vi "Analyze_Data.vi"(8 "error in (no error)":errorcluster, 9 "Number of Samples":dbl, 11 "Data In":dbl[](array[numeric])) -> (0 "error out":errorcluster)   [LabVIEW 2024]
uses:
  <vilib>/Analysis/2dsp.llb/Real FFT.vi
  <vilib>/Analysis/NI_AALPro.lvlib
  <vilib>/Analysis/NI_AALBase.lvlib
panel:
  in  "Copy Graph Data (Mag)":bool
  in  "Copy Graph Data (Phase)":bool
  out "Phase Spectrum":dbl[](graph) caption="Magnitude Spectrum"
  in  "Copy Graph Phase":bool
  in  "Copy Graph (Mag)":bool
  out "Amplitude":string
  out "Frequency (Hz)":string
  in  "Annotate List Cluster":T1
  in  "Show Labels":bool
  in  "Voltage Analysis":bool
  out "Output 2":string
  out "Output":string
  in  "FFT Analysis":bool
  in  "Statistic Analysis":bool
  out "Magnitude Spectrum":dbl[](graph)
  # "Frequency Peaks:"
  # "Frequency (Hz)"
  # "Amplitude"
  # "F0\nF1\nF2"
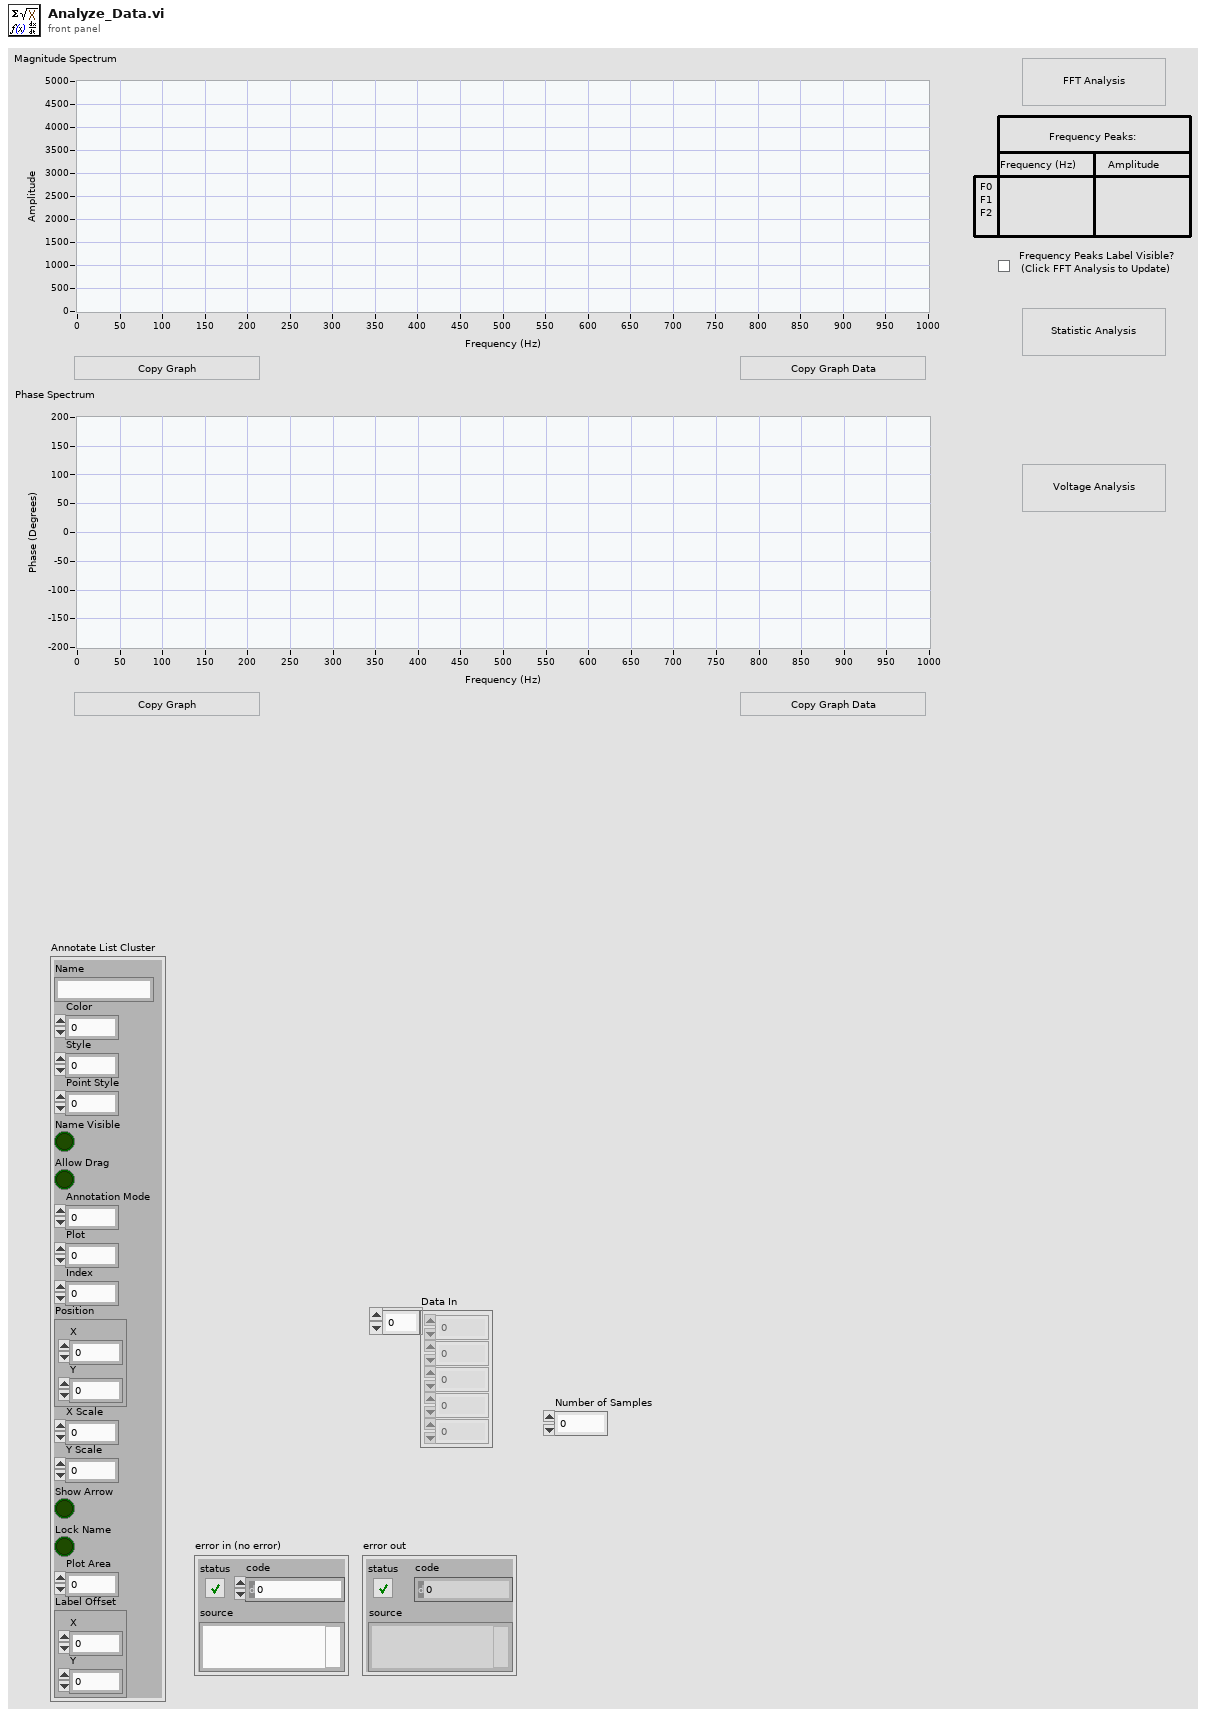
[diagram p1: front panel]
types:
  T1 = cluster{"Name":string, "Color":u32, "Style":u8, "Point Style":u8, "Name Visible":bool, "Allow Drag":bool, "Annotation Mode":u32, "Plot":i32, "Index":i32, "Position":cluster{"X":dbl, "Y":dbl}, "X Scale":u32, "Y Scale":u32, "Show Arrow":bool, "Lock Name":bool, "Plot Area":i32, "Label Offset":cluster{"X":dbl, "Y":dbl}}
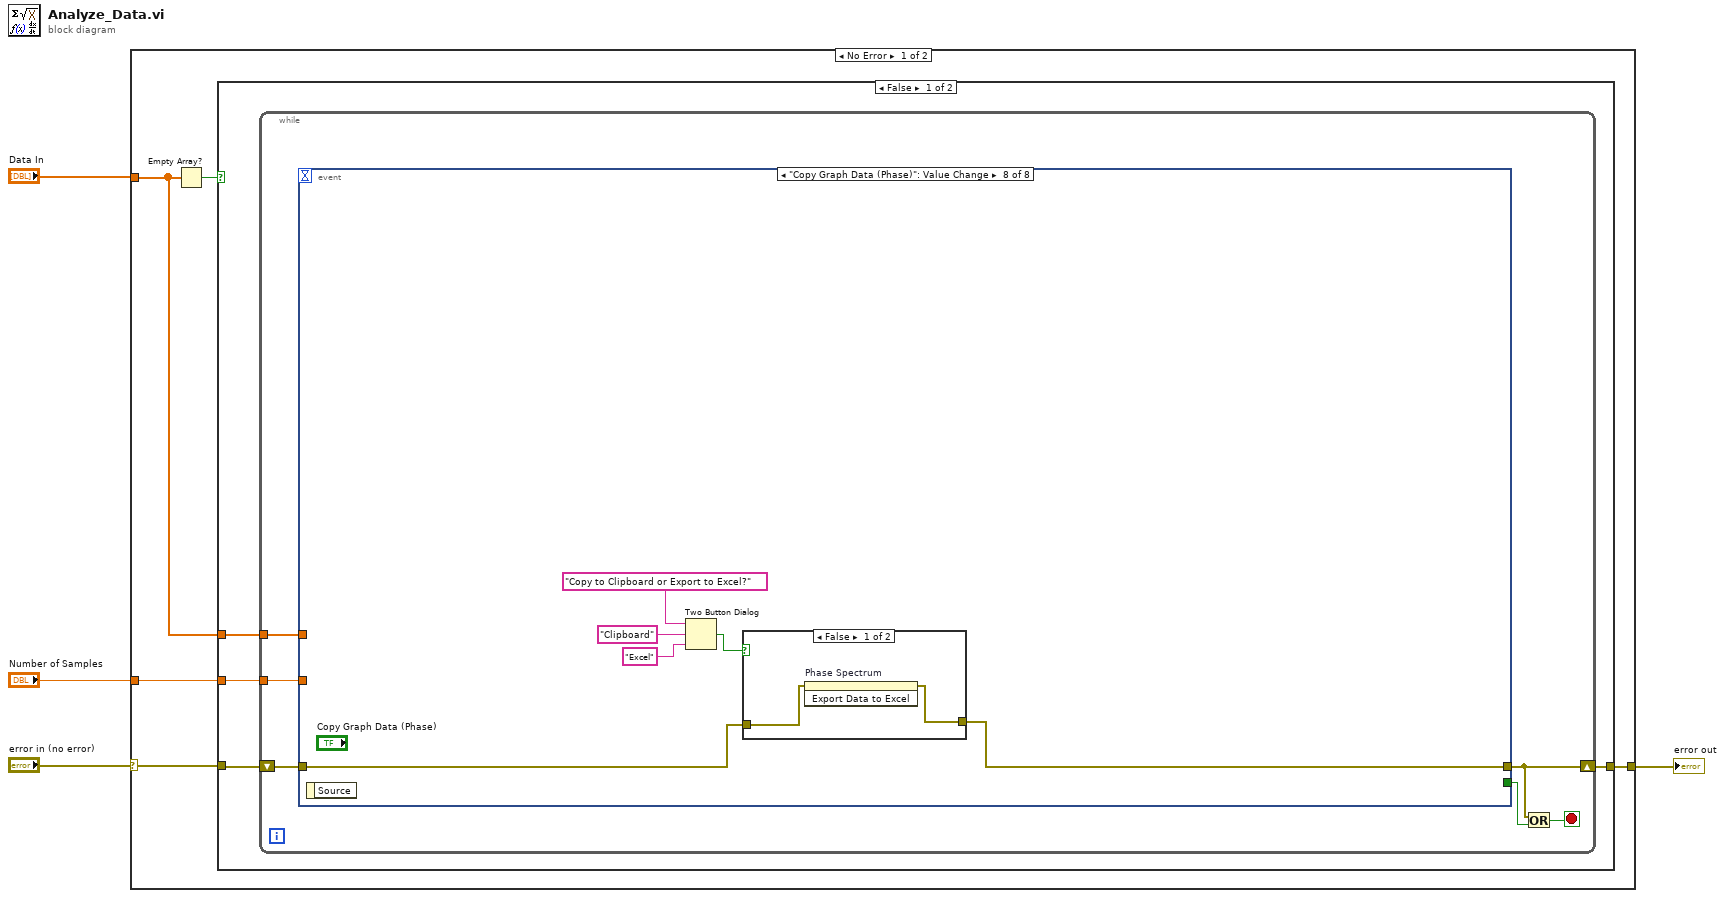
[diagram p0: block diagram]
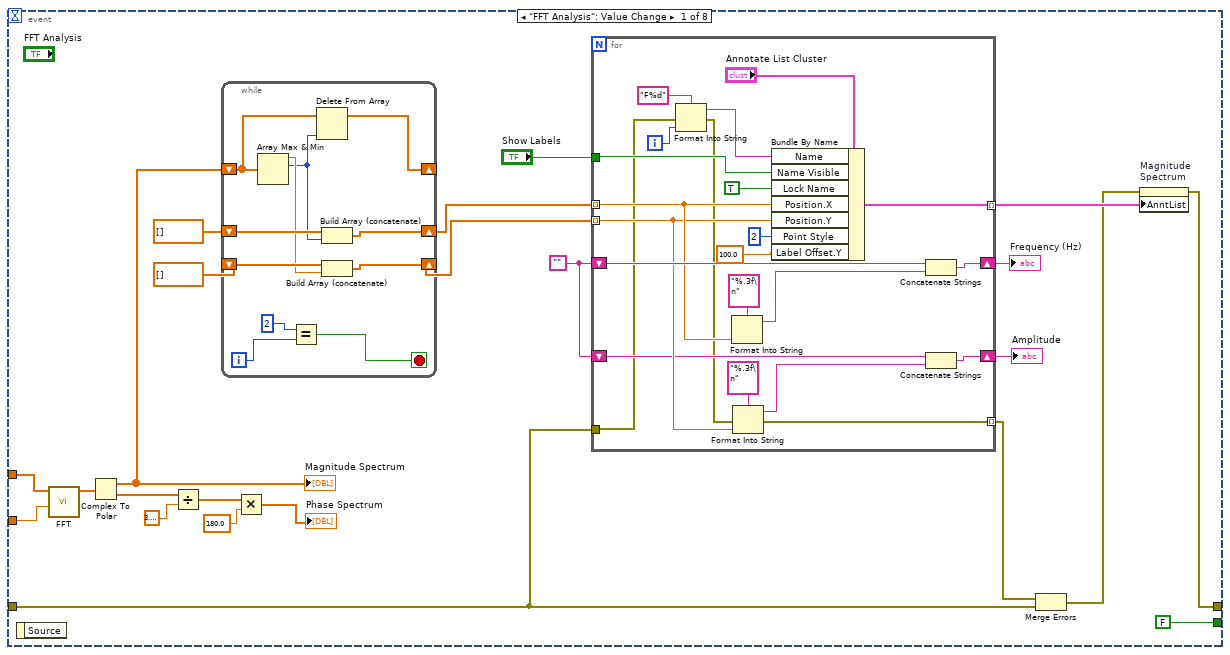
[diagram p2: hidden frame]
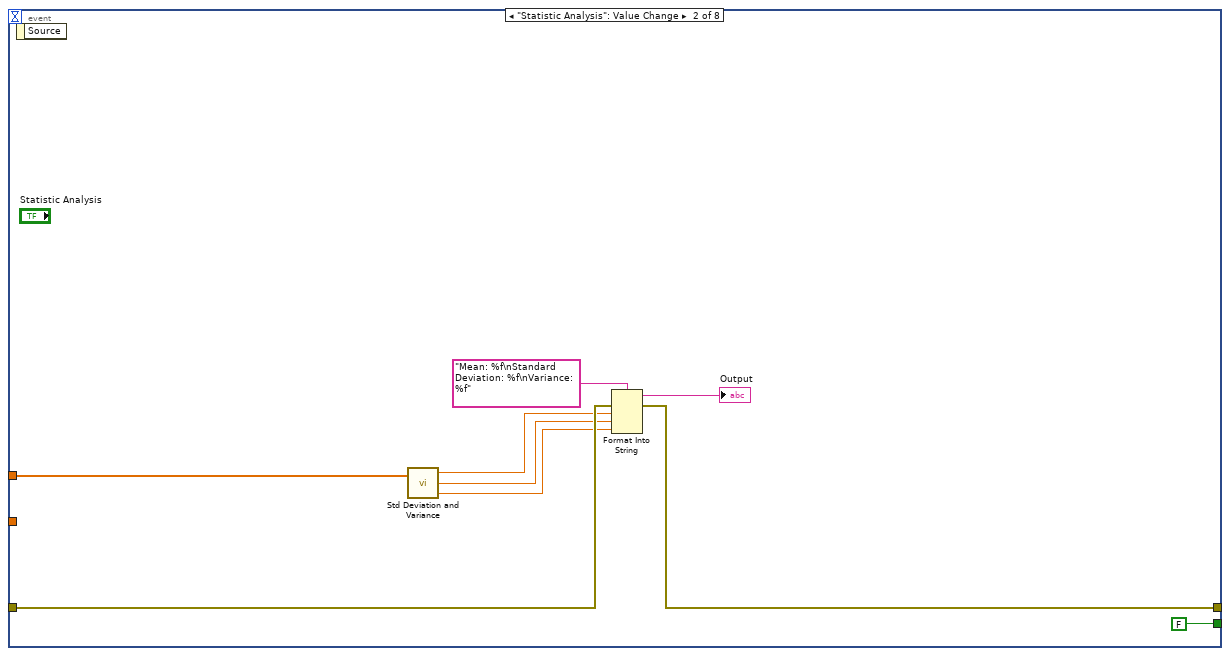
[diagram p3: hidden frame]
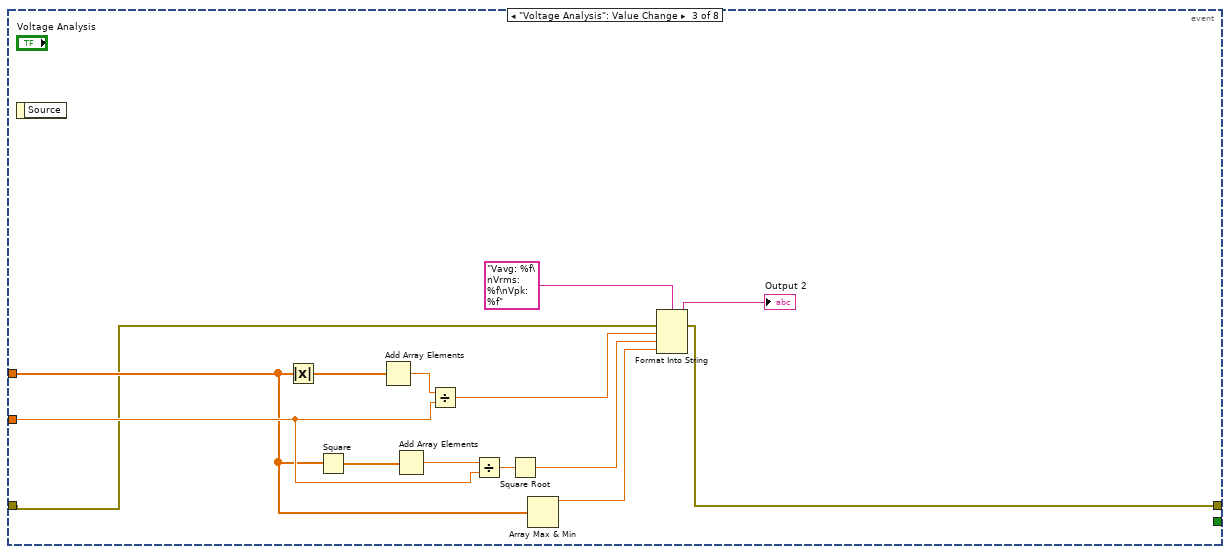
[diagram p4: hidden frame]
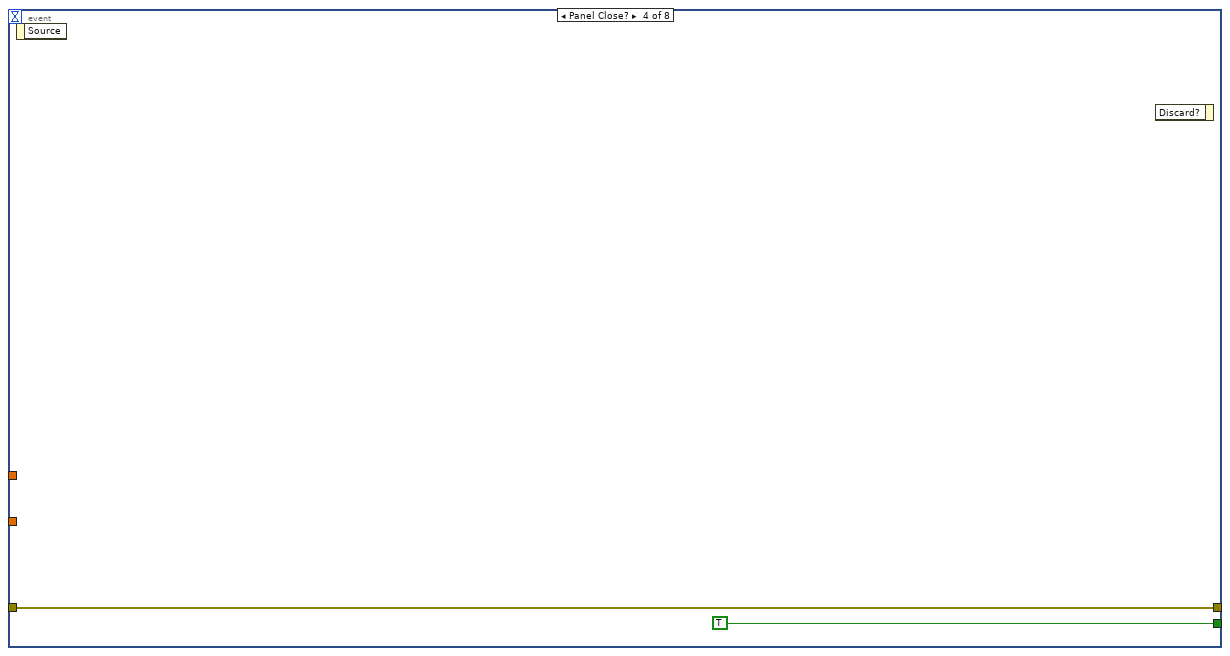
[diagram p5: hidden frame]
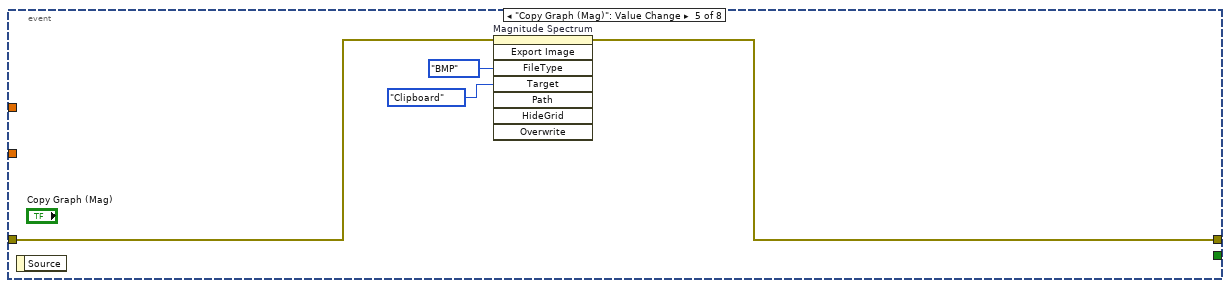
[diagram p6: hidden frame]
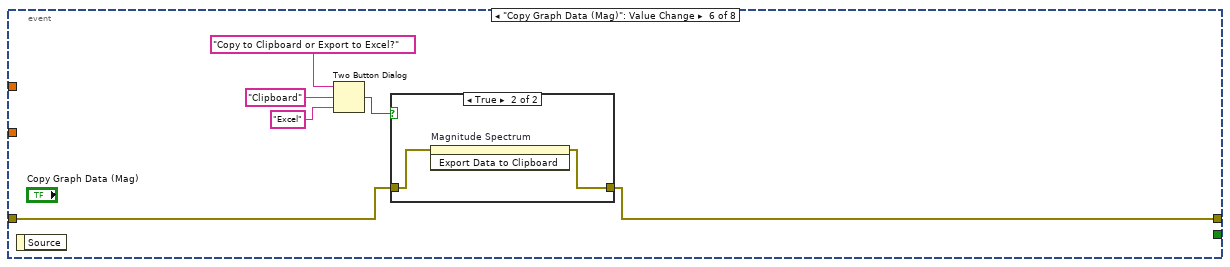
[diagram p7: hidden frame]
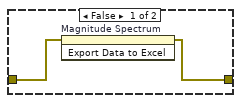
[diagram p8: hidden frame]
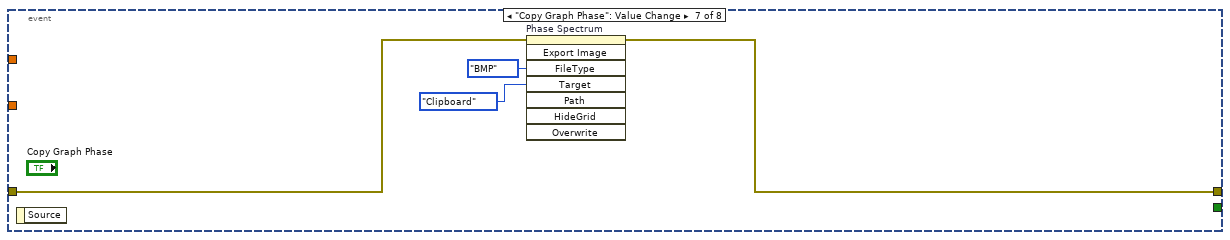
[diagram p9: hidden frame]
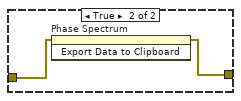
[diagram p10: hidden frame]
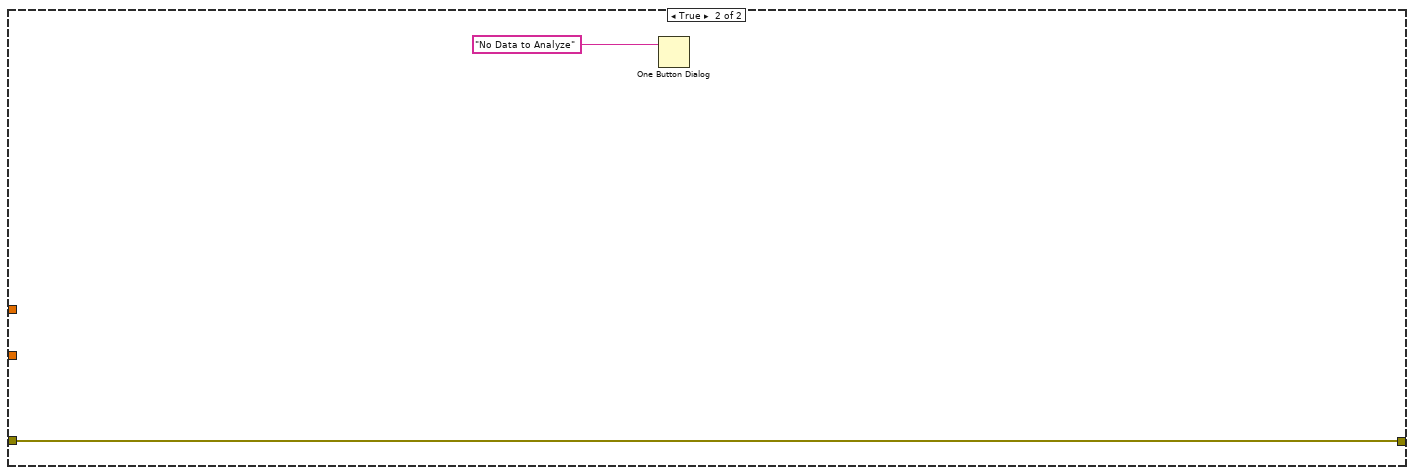
[diagram p11: hidden frame]
diagram:
  n1 = case shown="No Error" "error in (no error)" {
    selector: "error in (no error)" -> [w7 w131]
    tunnel: "Data In" -> [w8 _]
    tunnel: [w5 w131] -> w2
    tunnel: "Number of Samples" -> [w6 _]
    frame No Error {
      n2 = Empty Array?(array=w8) -> (empty?=w9:bool)
      n3 = case shown="False" w9 {
        tunnel: w8 -> [w11 _]
        tunnel: w7 -> [w13 w130]
        tunnel: [w12 w130] -> w5
        tunnel: w6 -> [w10 _]
        frame False {
          n4 = while {
            tunnel: w11 -> [w18]
            tunnel: w10 -> [w17]
            shift-right: [w15] -> w12
            shift-left: w13 -> [w19]
            stop <- w14 stop-if-true
            n5 = event shown="[7] \"Copy Graph Data (Phase)\": Value Change" {
              selector: _ -> [_ _ _ _ _ _ _ _]
              dyn-events: _ -> [_ _ _ _ _ _ _ _]
              timeout: _ -> [_ _ _ _ _ _ _ _]
              tunnel: w19 -> [w22 w82 w86 w99 w104 w107 w118 w121]
              tunnel: [w20 w83 w85 w99 w103 w106 w117 w119] -> w15
              tunnel: w18 -> [w33 w79 w87 _ _ _ _ _]
              tunnel: w17 -> [w37 _ w93 _ _ _ _ _]
              tunnel: [FALSE FALSE _ TRUE _ _ _ _] -> w16
              event "FFT Analysis": Value Change {
                w26 = ""
                n6 = event-data() -> ()  [unwired: 1 in, 1 out]
                n7 = call-poly <vilib>:"FFT.vi"("FFT size"=w37, "X"=w33) -> ("FFT {X}"=w42:cdb[])  [unwired: 8 in, 1 out]
                n8 = Complex To Polar(r * e^(i*theta)=w42) -> (r=w28:dbl[], theta=w38:dbl[])
                "Magnitude Spectrum" <- w28
                n9 = Divide(x=w38, y=3.141592653589793) -> (x/y=w40:dbl[])
                n10 = while {
                  shift-right: [w52] -> _
                  shift-left: w28 -> [w53]
                  shift-right: [w46] -> w30
                  shift-left: dbl[] [] ("Data In") -> [w51]
                  shift-right: [w49] -> w29
                  shift-left: dbl[] [] ("Data In") -> [w50]
                  i -> [w45]
                  stop <- w43 stop-if-true
                  n11 = Array Max & Min(array=w53) -> (max value=w48:dbl, max index (indices)=w47:i32)  [unwired: 2 out]
                  n12 = Equal?(x=2, y=w45) -> (x = y?=w43:bool)
                  n13 = Delete From Array(array=w53, index=w47) -> (array with subset deleted=w52:dbl[])  [unwired: 1 in, 1 out]
                  n14 = Build Array (concatenate)(w51, w47) -> (w46:dbl[])
                  n15 = Build Array (concatenate)(w50, w48) -> (w49:dbl[])
                }
                n16 = Multiply(x=w40, y=180.0) -> (x*y=→"Phase Spectrum":dbl[])
                n17 = for {
                  tunnel: "Show Labels" -> [w72]
                  tunnel: [w71] -> w34 mode=indexing
                  tunnel: w29 -> [w64] mode=indexing
                  tunnel: w30 -> [w65] mode=indexing
                  shift-right: [w69] -> w27
                  shift-left: w26 -> [w68]
                  shift-right: [w61] -> w25
                  shift-left: w26 -> [w62]
                  tunnel: w22 -> [w55]
                  tunnel: [w54] -> w23 mode=indexing
                  i -> [w59]
                  n18 = Format Into String(format string="F%d", error in=w55, w59) -> (resulting string=w74:string, error out=w56:errorcluster)  [unwired: 1 in]
                  n19 = Format Into String(format string="%.3f\n", w65) -> (resulting string=w63:string)  [unwired: 2 in, 1 out]
                  n20 = Format Into String(format string="%.3f\n", error in=w56, w64) -> (resulting string=w60:string, error out=w54:errorcluster)  [unwired: 1 in]
                  n21 = Bundle By Name(cluster="Annotate List Cluster", "Name"=w74, "Name Visible"=w72, "Lock Name"=TRUE ("Name Visible"), "Position.X"=w65, "Position.Y"=w64, "Point Style"=u8 2, "Label Offset.Y"=100.0) -> (w71:T1)
                  n22 = Concatenate Strings(w68, w63) -> (w69:string)
                  n23 = Concatenate Strings(w62, w60) -> (w61:string)
                }
                "Frequency (Hz)" <- w27
                "Amplitude" <- w25
                n24 = Merge Errors(w23, w22) -> (w21:errorcluster)
                n25 = property on="Magnitude \nSpectrum" class="WFGraph (strict)"(error in=w21, "AnntList"=w34) -> (error out=w20:errorcluster)  [unwired: 1 in, 1 out]
              }
              event "Statistic Analysis": Value Change {
                n26 = event-data() -> ()  [unwired: 1 in, 1 out]
                n27 = call <vilib>:"Std Deviation and Variance.vi"("X"=w79) -> ("mean"=w78:dbl, "standard deviation"=w77:dbl, "variance"=w76:dbl)  [unwired: 1 in]
                n28 = Format Into String(format string="Mean: %f\nStandard Deviation: %f\nVariance: %f" ("initial string"), error in=w82, w78, w77, w76) -> (resulting string=→"Output":string, error out=w83:errorcluster)  [unwired: 1 in]
              }
              event "Voltage Analysis": Value Change {
                n29 = event-data() -> ()  [unwired: 1 in, 1 out]
                n30 = Absolute Value(x=w87) -> (abs(x)=w97:dbl[])
                n31 = Square(x=w87) -> (x^2=w95:dbl[])
                n32 = Add Array Elements(numeric array=w97) -> (sum=w98:dbl)
                n33 = Add Array Elements(numeric array=w95) -> (sum=w94:dbl)
                n34 = Divide(x=w98, y=w93) -> (x/y=w96:dbl)
                n35 = Divide(x=w94, y=w93) -> (x/y=w92:dbl)
                n36 = Square Root(x=w92) -> (sqrt(x)=w91:dbl)
                n37 = Array Max & Min(array=w87) -> (max value=w90:dbl)  [unwired: 3 out]
                n38 = Format Into String(format string="Vavg: %f\nVrms: %f\nVpk: %f" ("initial string"), error in=w86, w96, w91, w90) -> (resulting string=→"Output 2":string, error out=w85:errorcluster)  [unwired: 1 in]
              }
              event Panel Close? {
                n39 = event-data() -> ()  [unwired: 1 in, 1 out]
                n40 = event-data() -> ()  [unwired: 2 in, 1 out]
              }
              event "Copy Graph (Mag)": Value Change {
                n41 = event-data() -> ()  [unwired: 1 in, 1 out]
                n42 = invoke on="Magnitude Spectrum" class="WFGraph (strict)" method="Export Image"(error in=w104, "FileType"=enum32{"BMP", "EPS", "EMF", "PICT"}."BMP" ("File Type"), "Target"=enum32{"File", "Clipboard"}."Clipboard") -> (error out=w103:errorcluster)  [unwired: 5 in, 7 out]
              }
              event "Copy Graph Data (Mag)": Value Change {
                n43 = event-data() -> ()  [unwired: 1 in, 1 out]
                n44 = Two Button Dialog(message="Copy to Clipboard or Export to Excel?", 1:"Excel" ("F button name (\"Cancel\")"), 2:"Clipboard" ("T button name (\"OK\")")) -> (T button?=w105:bool)
                n45 = case shown="True" w105 {
                  tunnel: w107 -> [w112 w114]
                  tunnel: [w111 w113] -> w106
                  frame False {
                    n46 = invoke on="Magnitude Spectrum" class="WFGraph (strict)" method="Export Data to Excel"(error in=w112) -> (error out=w111:errorcluster)  [unwired: 2 in, 2 out]
                  }
                  frame True {
                    n47 = invoke on="Magnitude Spectrum" class="WFGraph (strict)" method="Export Data to Clipboard"(error in=w114) -> (error out=w113:errorcluster)  [unwired: 2 in, 2 out]
                  }
                }
              }
              event "Copy Graph Phase": Value Change {
                n48 = event-data() -> ()  [unwired: 1 in, 1 out]
                n49 = invoke on="Phase Spectrum" class="WFGraph (strict)" method="Export Image"(error in=w118, "FileType"=enum32{"BMP", "EPS", "EMF", "PICT"}."BMP" ("File Type"), "Target"=enum32{"File", "Clipboard"}."Clipboard") -> (error out=w117:errorcluster)  [unwired: 5 in, 7 out]
              }
              event "Copy Graph Data (Phase)": Value Change {
                n50 = event-data() -> ()  [unwired: 1 in, 1 out]
                n51 = Two Button Dialog(message="Copy to Clipboard or Export to Excel?", 1:"Excel" ("F button name (\"Cancel\")"), 2:"Clipboard" ("T button name (\"OK\")")) -> (T button?=w120:bool)
                n52 = case shown="False" w120 {
                  tunnel: w121 -> [w126 w127]
                  tunnel: [w125 w128] -> w119
                  frame False {
                    n53 = invoke on="Phase Spectrum" class="WFGraph (strict)" method="Export Data to Excel"(error in=w126) -> (error out=w125:errorcluster)  [unwired: 2 in, 2 out]
                  }
                  frame True {
                    n54 = invoke on="Phase Spectrum" class="WFGraph (strict)" method="Export Data to Clipboard"(error in=w127) -> (error out=w128:errorcluster)  [unwired: 2 in, 2 out]
                  }
                }
              }
            }
            n55 = Or(x=w15, y=w16) -> (x .or. y?=w14:bool)
          }
        }
        frame True {
          n56 = One Button Dialog(message="No Data to Analyze") -> ()  [unwired: 1 in, 1 out]
        }
      }
    }
    frame Error {
    }
  }
  "error out" <- w2
